vi "test_libssh2_hostkey_hash.vi"() -> ()   [LabVIEW 2013, in "libssh2_integration_tests.lvlib"]
uses:
  libssh2_integration_tests.lvlib
  libssh2/Host Key Hash Type.ctl
  <vilib>/addons/_JKI Toolkits/Caraya/classes/Test/Test.lvclass
  <vilib>/addons/_JKI Toolkits/Caraya/classes/Assert/Assert.lvclass
  libssh2/libssh2.lvlib
panel:
  out "error out":errorcluster
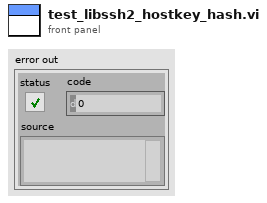
[diagram p1: front panel]
types:
  T1 = typedef "libssh2.lvlib/Host Key Hash Type.ctl" = enum16{"MD5", "SHA1", "SHA256"}
  T2 = typedef "libssh2.lvlib/Session Refnum.ctl" = refnum<k1>
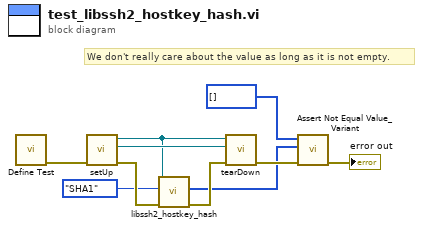
[diagram p0: block diagram]
diagram:
  # "We don't really care about the value as long as it is not empty."
  n1 = call <vilib>:"Define Test.vi"() -> ("error out"=w10:errorcluster)  [unwired: 10 in, 1 out]
  n2 = call "setUp.vi"("error in (no error)"=w10) -> ("error out"=w6:errorcluster, "connection ID"=w9:refnum<k5>, "session"=w8:T2)  [unwired: 8 in]
  n3 = call "libssh2_hostkey_hash.vi"("error in (no error)"=w6, "hash type"=Host_Key_Hash_Type."SHA1", "session"=w8) -> ("error out"=w7:errorcluster, "hash"=w1:u8[])  [unwired: 7 in]
  n4 = call "tearDown.vi"("error in (no error)"=w7, "connection ID"=w9, "session"=w8) -> ("error out"=w5:errorcluster)  [unwired: 8 in]
  n5 = call <vilib>:"Assert Not Equal Value_Variant.vi"("error in (no error)"=w5, "Y"=w1, "X"=u8[] []) -> ("error out"=→"error out":errorcluster)  [unwired: 7 in, 1 out]
